vi "PluginTemplate.vi"(1 "ServerPort":i32, 2 "ServerName":string) -> ()   [LabVIEW 2014]
doc: "Use this template to build a standard state machine design pattern. Each state executes code and determines which state to transition to. Contrast this design pattern with the user interface event pattern, in which code executes in response to user actions. Contrast this design pattern also with the queued message handler pattern, in which each message handling code can queue zero or more new messages."
panel:
  in  "Close":bool
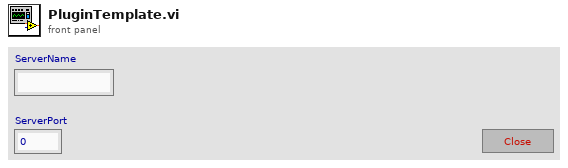
[diagram p1: front panel]
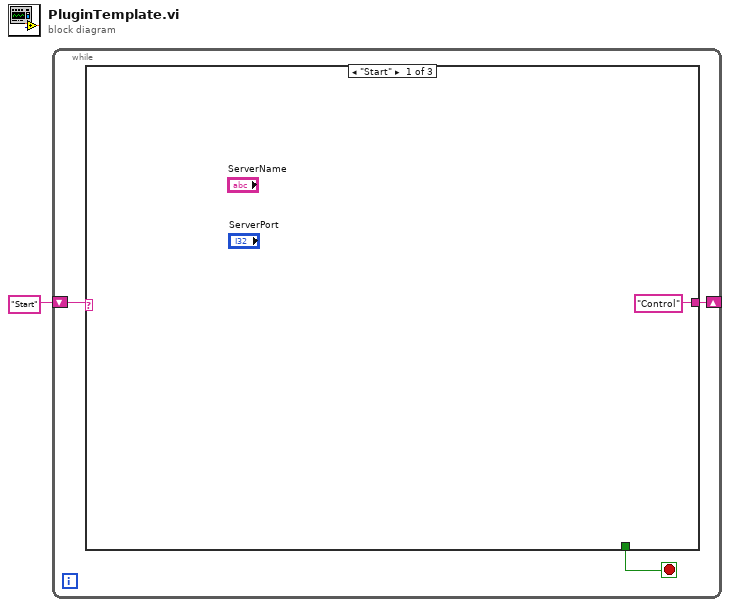
[diagram p0: block diagram]
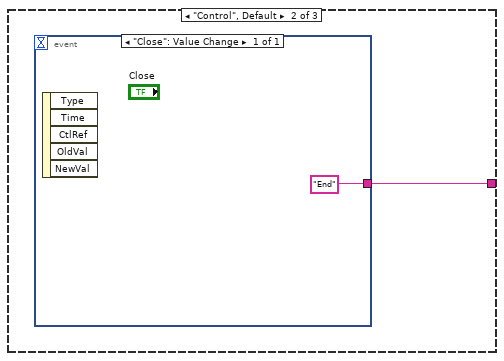
[diagram p2: hidden frame]
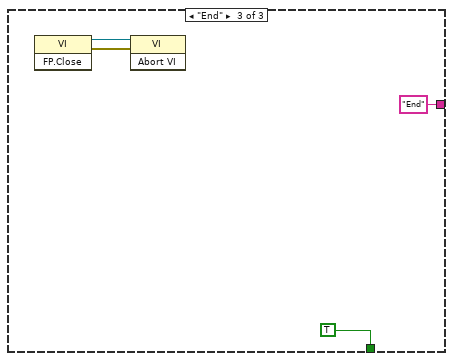
[diagram p3: hidden frame]
diagram:
  n1 = while {
    shift-right: [w3] -> _
    shift-left: "Start" -> [w4]
    stop <- w2 stop-if-true
    n2 = case shown="\"Start\"" w4 {
      tunnel: ["Control" w6 "End"] -> w3
      tunnel: [_ _ TRUE] -> w2
      frame "Start" {
      }
      frame "Control", Default {
        n3 = event shown="[0] \"Close\": Value Change" {
          selector: _ -> [_]
          dyn-events: _ -> [_]
          timeout: _ -> [_]
          tunnel: ["End"] -> w6
          event "Close": Value Change {
            n4 = event-data() -> ()  [unwired: 1 in, 5 out]
          }
        }
      }
      frame "End" {
        n5 = invoke class="VI" method="FP.Close"() -> (reference out=w8:refnum<vi>, error out=w9:errorcluster)  [unwired: 3 in, 1 out]
        n6 = invoke class="VI" method="Abort VI"(reference=w8, error in=w9) -> ()  [unwired: 1 in, 3 out]
      }
    }
  }
